vi "check_robot.vi"() -> ()   [LabVIEW 2026]
panel:
  out "Array 2":string[](array[string])
  out "result":bool
  in  "Array":string[](array[string])
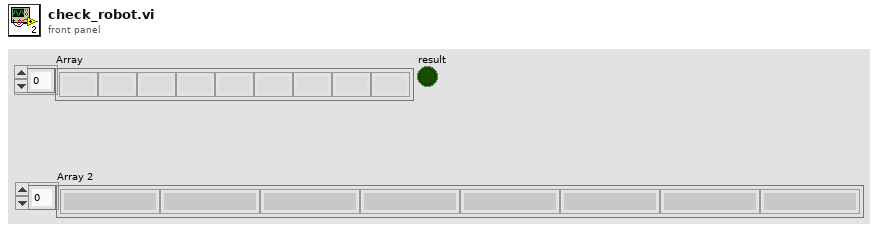
[diagram p1: front panel]
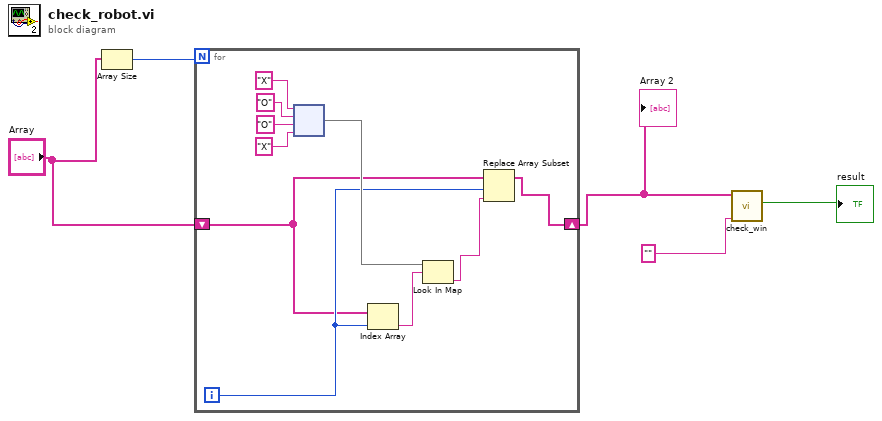
[diagram p0: block diagram]
diagram:
  n1 = Array Size(array="Array") -> (size(s)=w4:i32)
  n2 = for {
    N: w4 -> [_]
    shift-right: [w6] -> w2
    shift-left: "Array" -> [w9]
    i -> [w10]
    n3 = node("X" ("key"), "O", "O", "X" ("key")) -> (w11:map{string, string})
    n4 = Index Array(array=w9, index=w10) -> (element=w8:string)
    n5 = Look In Map(map=w11, key=w8) -> (value=w7:string)  [unwired: 1 in, 1 out]
    n6 = Replace Array Subset(array=w9, new element=w7, index=w10) -> (w6:string[])
  }
  "Array 2" <- w2
  n7 = call "check_win.vi"("check against"="", "Array"=w2) -> ("result"=→"result":bool)  [unwired: 9 in]
